vi "Write Configuration.vi"(8 "error in (no error)":errorcluster, 10 "Configuration":T1, 11 "RandomNumberGenerator Controller in":refnum<class "RandomNumberGenerator Controller.lvclass">) -> (0 "error out":errorcluster, 3 "RandomNumberGenerator Controller out":refnum<class "RandomNumberGenerator Controller.lvclass">)   [LabVIEW 2020, in "RandomNumberGenerator.lvlib" / "RandomNumberGenerator Controller.lvclass"]
doc: "<b>Write Configuration</b>\nWrites the configuration information to the plugin controller class data."
uses:
  RandomNumberGenerator Controller.lvclass
  RandomNumberGenerator Controller.lvclass/RandomNumberGenerator Controller.ctl
  PE/Configuration.ctl
  PE/RandomNumberGenerator.lvclass
panel:
  # "#via_ignore"
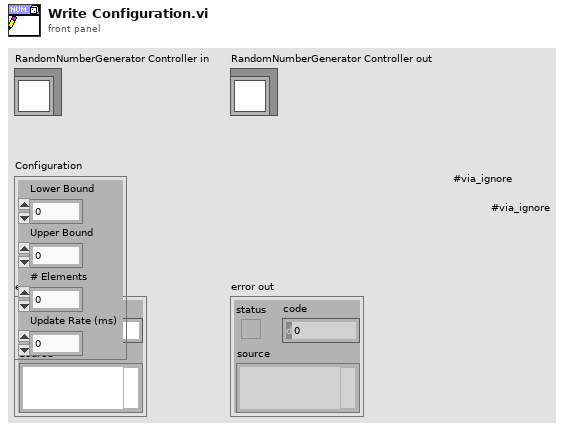
[diagram p1: front panel]
types:
  T1 = typedef "RandomNumberGenerator.lvlib/RandomNumberGenerator.lvclass/Configuration.ctl" = cluster{"Lower Bound":dbl, "Upper Bound":dbl, "# Elements":i32, "Update Rate (ms)":i32}
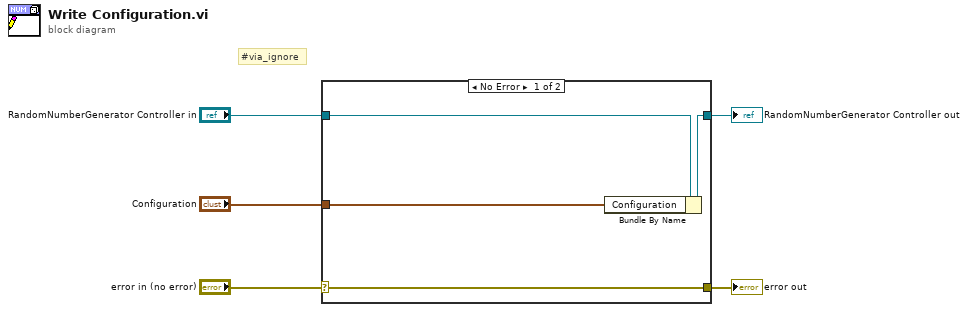
[diagram p0: block diagram]
diagram:
  # "#via_ignore"
  n1 = case shown="No Error" "error in (no error)" {
    selector: "error in (no error)" -> [w9 w10]
    tunnel: [w9 w10] -> w4
    tunnel: [w7 w11] -> w2
    tunnel: "RandomNumberGenerator Controller in" -> [w8 w11]
    tunnel: "Configuration" -> [w6 _]
    frame No Error {
      n2 = Bundle By Name(cluster=w8, "Configuration"=w6) -> (w7:refnum<class "RandomNumberGenerator Controller.lvclass">)
    }
    frame Error {
    }
  }
  "error out" <- w4
  "RandomNumberGenerator Controller out" <- w2
